vi "例4.14通知型事件和过滤型事件的区别.vi"() -> ()   [LabVIEW 2017]
panel:
  in  "停止":bool
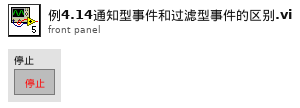
[diagram p1: front panel]
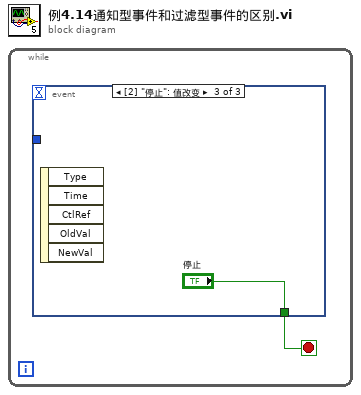
[diagram p0: block diagram]
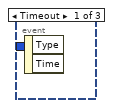
[diagram p2: hidden frame]
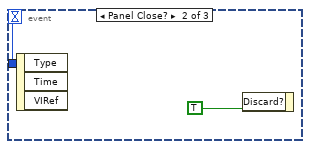
[diagram p3: hidden frame]
diagram:
  n1 = while {
    stop <- w1 stop-if-true
    n2 = event shown="[2] \"停止\": 值改变" {
      selector: _ -> [_ _ _]
      dyn-events: _ -> [_ _ _]
      timeout: _ -> [_ w3 _]
      tunnel: [_ _ "停止"] -> w1
      tunnel: [_ w3 _] -> _
      event Timeout {
        n3 = event-data() -> ()  [unwired: 1 in, 2 out]
      }
      event Panel Close? {
        n4 = event-data() -> ()  [unwired: 1 in, 3 out]
        n5 = event-data("Discard?"=TRUE ("放弃？")) -> ()  [unwired: 1 in, 1 out]
      }
      event "停止": Value Change {
        n6 = event-data() -> ()  [unwired: 1 in, 5 out]
      }
    }
  }
